vi "Shut Down Device.vi"(8 "error in (no error)":errorcluster, 11 "Stage Controller in":refnum<class "Stage Controller.lvclass">) -> (0 "error out":errorcluster, 3 "Stage Controller out":refnum<class "Stage Controller.lvclass">)   [LabVIEW 2018, in "Stage Controller.lvlib" / "Stage Controller.lvclass"]
uses:
  Stage Controller.lvclass
  Stage Controller.lvclass/Stage Controller.ctl
  Device/Device.lvclass
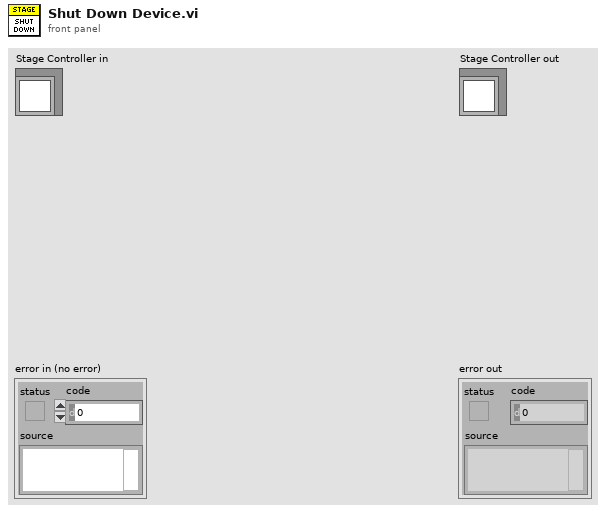
[diagram p1: front panel]
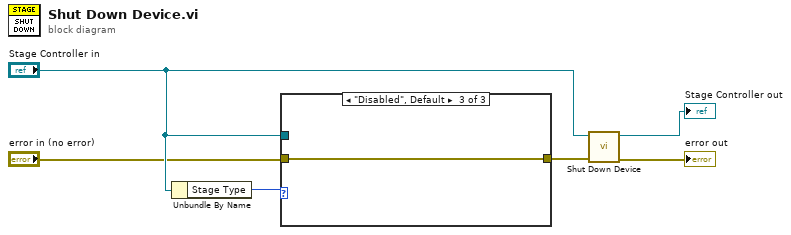
[diagram p0: block diagram]
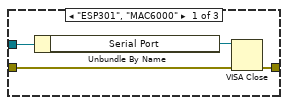
[diagram p2: hidden frame]
diagram:
  n1 = Unbundle By Name("Stage Controller in") -> ("Stage Type"=w4:enum16{"Disabled", "ESP301", "Ti2", "MAC6000"})
  n2 = case shown="\"Disabled\", Default" w4 {
    tunnel: "Stage Controller in" -> [w9 _ _]
    tunnel: "error in (no error)" -> [w8 w11 w12]
    tunnel: [w7 w11 w12] -> w1
    frame "ESP301", "MAC6000" {
      n3 = Unbundle By Name(w9) -> ("Serial Port"=w10:refnum<visa-resource-name>)
      n4 = VISA Close(VISA resource name=w10, error in (no error)=w8) -> (error out=w7:errorcluster)
    }
    frame "Ti2" {
    }
    frame "Disabled", Default {
    }
  }
  n5 = call-parent "Shut Down Device.vi"("error in (no error)"=w1, "Device in"="Stage Controller in") -> ("error out"=→"error out":errorcluster, "Device out"=→"Stage Controller out":refnum<class "Stage Controller.lvclass">)  [unwired: 8 in]
